vi "test Initialize and Finalize Hardware.vi"(8 "error in":errorcluster, 11 "test case in":refnum<class "Hardware API.lvclass">) -> (0 "error out":errorcluster, 3 "test case out":refnum<class "Hardware API.lvclass">)   [LabVIEW 2020, in "Hardware API.lvclass"]
uses:
  Hardware API.lvclass
  <vilib>/addons/_JKI Toolkits/VI Tester/TestCase.llb/TestCase.lvclass
  Hardware API/AIM ARINC 429 Hardware API.lvlib
  C:/Program Files (x86)/National Instruments/LabVIEW 2020/vi.lib/addons/_JKI Toolkits/VI Tester/TestCase.llb/TestCase.lvclass
  C:/Git/niveristand-aim-arinc429-custom-device/Source/Custom Device Support/Tests/Unit/Hardware API/Hardware API.lvclass
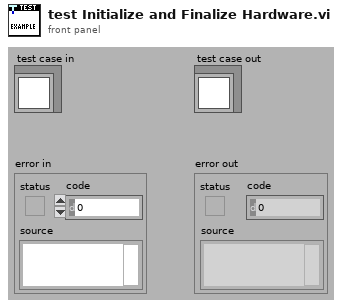
[diagram p1: front panel]
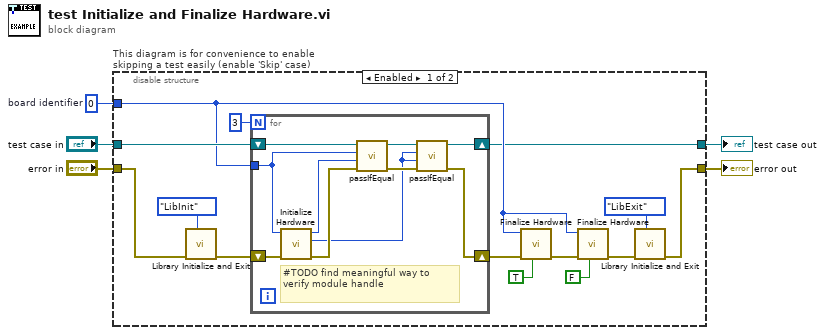
[diagram p0: block diagram]
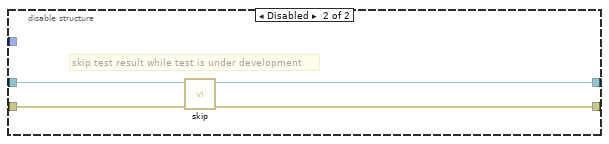
[diagram p2: hidden frame]
diagram:
  w1 = u8 0  # board identifier
  n1 = disable-structure "This diagram is for convenience to enable skipping a test easily (enable 'Skip' case)" shown="Enabled" {
    disable-tunnel: "test case in" -> [w19 w33]
    disable-tunnel: [w7 w31] -> w2
    disable-tunnel: [w15 w32] -> w4
    disable-tunnel: "error in" -> [w18 w30]
    disable-tunnel: w1 -> [w10 _]
    frame Enabled {
      n2 = call "Library Initialize and Exit.vi"("action"=enum16{"LibInit", "LibExit"}."LibInit", "error in"=w18) -> ("error out"=w14:errorcluster)  [unwired: 7 in, 2 out]
      n3 = for {
        N: 3 -> [_]
        shift-right: [w26] -> w7
        shift-left: w19 -> [w29]
        shift-right: [w23] -> w13
        shift-left: w14 -> [w25]
        tunnel: w10 -> [w22]
        # "#TODO find meaningful way to verify module handle"
        n4 = call "Initialize Hardware.vi"("error in"=w25, "board identifier in"=w22) -> ("error out"=w24:errorcluster, "module handle out"=w21:u8, "board identifier out"=w20:u8)  [unwired: 7 in]
        n5 = call-dynamic "passIfEqual.vi"("error in (no error)"=w24, "y"=w20, "x"=w22, "TestCase in"=w29) -> ("error out"=w27:errorcluster, "TestCase out"=w28:refnum<class "Hardware API.lvclass">)  [unwired: 6 in]
        n6 = call-dynamic "passIfEqual.vi"("error in (no error)"=w27, "y"=w21, "x"=w21, "TestCase in"=w28) -> ("error out"=w23:errorcluster, "TestCase out"=w26:refnum<class "Hardware API.lvclass">)  [unwired: 6 in]
      }
      n7 = call "Finalize Hardware.vi"("force (F)"=TRUE, "error in"=w13, "board identifier"=w10) -> ("error out"=w9:errorcluster)  [unwired: 8 in]
      n8 = call "Finalize Hardware.vi"("force (F)"=FALSE, "error in"=w9, "board identifier"=w10) -> ("error out"=w6:errorcluster)  [unwired: 8 in]
      n9 = call "Library Initialize and Exit.vi"("action"=enum16{"LibInit", "LibExit"}."LibExit", "error in"=w6) -> ("error out"=w15:errorcluster)  [unwired: 7 in, 2 out]
    }
    frame Disabled {
      # "skip test result while test is under development"
      n10 = call <vilib>:"skip.vi"("error in (no error)"=w30, "TestCase in"=w33) -> ("error out"=w32:errorcluster, "TestCase out"=w31:refnum<class "Hardware API.lvclass">)  [unwired: 8 in]
    }
  }
  "error out" <- w4
  "test case out" <- w2
